vi "publish -- pick nameed element.vi"(9 "name":string="dlogR/dlogT -- S", 10 "nanocal data array":T1[](array[typedef])=[{"name"="dlogR/dlogT -- S ", "units"="aaa", "data"=0.2}, {"name"="Ts", "units"="K", "data"=9.0}]) -> (1 "element":dbl, 2 "nanocal data array OUT":T1[](array[typedef])=[{"name"="dlogR/dlogT -- S ", "units"="aaa", "data"=0.2}, {"name"="Ts", "units"="K", "data"=9.0}])   [LabVIEW 2018]
uses:
  icicle.ctl
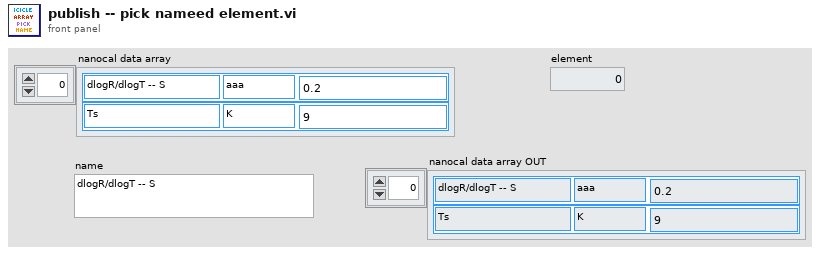
[diagram p1: front panel]
types:
  T1 = typedef "icicle.ctl" = cluster{"name":string, "units":string, "data":dbl}
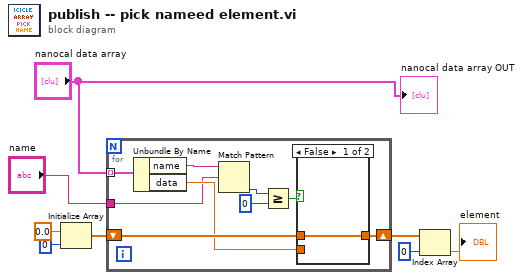
[diagram p0: block diagram]
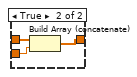
[diagram p2: hidden frame]
diagram:
  n1 = Initialize Array(0.0 ("element"), 0 ("dimension size")) -> (w6:dbl[])
  n2 = for {
    tunnel: "nanocal data array" -> [w17] mode=indexing
    shift-right: [w12] -> w5
    shift-left: w6 -> [w13]
    tunnel: "name" -> [w9]
    n3 = Unbundle By Name(w17) -> ("name"=w16:string, "data"=w11:dbl)
    n4 = Match Pattern(string=w16, regular expression=w9) -> (offset past match=w15:i32)  [unwired: 1 in, 3 out]
    n5 = Greater Or Equal?(x=w15, y=0) -> (x >= y?=w10:bool)
    n6 = case shown="False" w10 {
      tunnel: w13 -> [w18 w21]
      tunnel: [w18 w20] -> w12
      tunnel: w11 -> [_ w19]
      frame False {
      }
      frame True {
        n7 = Build Array (concatenate)(w21, w19) -> (w20:dbl[])
      }
    }
  }
  n8 = Index Array(array=w5, index=0) -> (element=→"element":dbl)
  "nanocal data array OUT" <- "nanocal data array"
